vi "PH_gentec_M-Link.set Enable Anticipation.vi"(0 "i ref in":refnum<vi>, 2 "VISA resource in":refnum<visa-resource-name>, 5 "error in":errorcluster) -> (11 "Timeout":bool, 13 "Data read":string[](array[string]), 14 "i ref out":refnum<vi>, 16 "VISA resource out":refnum<visa-resource-name>, 17 "Error":bool, 18 "Failure":bool, 19 "error out":errorcluster)   [LabVIEW 2014, in "PH_gentec_M-Link.lvlib"]
doc: "This VI writes wanted Settings to the Device and checks the result."
uses:
  PH_gentec_M-Link.lvlib
  non_GPL/instr.lib/gentec-M-LINK/gentec-M-Link - Driver.lvlib
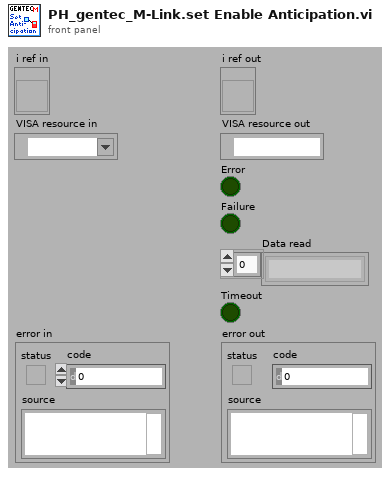
[diagram p1: front panel]
types:
  T1 = typedef "PH_gentec_M-Link.lvlib/PH_gentec_M-Link.i attribute.ctl" = cluster{"GUI References":cluster{"Wanted Head Settings":refnum<vi>, "Current Head Settings":refnum<vi>, "Set Auto Range":refnum<vi>, "Trigger Polarity":refnum<vi>, "Trigger Source":refnum<vi>, "Waveform Averages":refnum<vi>, "Continuous":refnum<vi>, "get one Value":refnum<vi>}, "Wanted Head Settings":T2, "Current Head Settings":T2}
  T2 = typedef "PH_gentec_M-Link.lvlib/PH_gentec_M-Link.Head Settings.ctl" = cluster{"Measurement Mode":T3, "Enable Anticipation":bool, "Set Auto Range":bool, "Block Signal":bool, "Set Head Attenuator":bool, "Enable SSE":bool, "Trigger Polarity":T4, "Trigger Source":T5, "Waveform Averages":T6, "Set Zero":i32, "Current Measurement":i32, "Start Data Flow":bool}
  T3 = typedef "gentec-M-Link - Driver.lvlib/gentec-M-Link.Measurement Mode.ctl" = u16
  T4 = typedef "gentec-M-Link - Driver.lvlib/gentec-M-Link.Trigger Polarity.ctl" = u16
  T5 = typedef "gentec-M-Link - Driver.lvlib/gentec-M-Link.Trigger Source.ctl" = u16
  T6 = typedef "gentec-M-Link - Driver.lvlib/gentec-M-Link.Waveform Averages.ctl" = u16
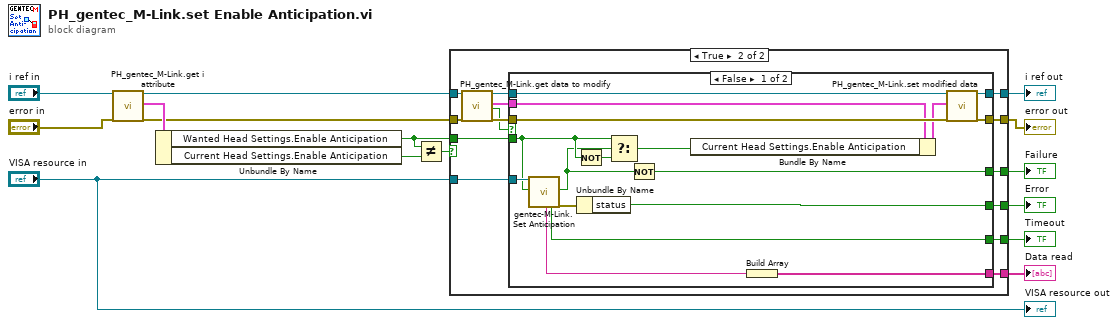
[diagram p0: block diagram]
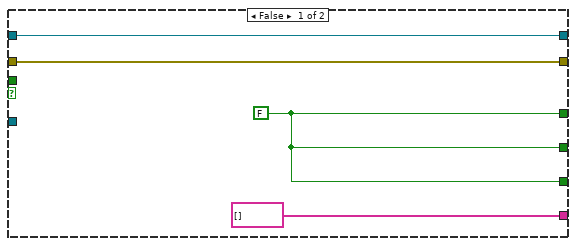
[diagram p2: hidden frame]
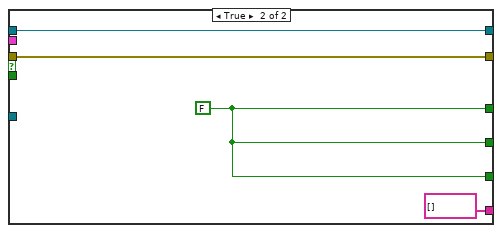
[diagram p3: hidden frame]
diagram:
  n1 = call "PH_gentec_M-Link.get i attribute.vi"("i ref in"="i ref in", "error in (no error)"="error in") -> ("i ref out"=w10:refnum<vi>, "i attribute"=w13:T1, "error out"=w12:errorcluster)  [unwired: 15 in]
  n2 = Unbundle By Name(w13) -> ("Wanted Head Settings.Enable Anticipation"=w6:bool, "Current Head Settings.Enable Anticipation"=w7:bool)
  n3 = Not Equal?(x=w6, y=w7) -> (x != y?=w5:bool)
  n4 = case shown="True" w5 {
    tunnel: [w18 w33] -> w15
    tunnel: [w19 w32] -> w14
    tunnel: w12 -> [w18 w27]
    tunnel: w10 -> [w19 w26]
    tunnel: "VISA resource in" -> [_ w25]
    tunnel: w6 -> [_ w24]
    tunnel: [w17 w23] -> w4
    tunnel: [w17 w22] -> w3
    tunnel: [w17 w21] -> w2
    tunnel: [string[] [] w20] -> w1
    frame False {
      w17 = FALSE
    }
    frame True {
      n5 = call "PH_gentec_M-Link.get data to modify.vi"("i ref in"=w26, "error in (no error)"=w27) -> ("i ref out"=w30:refnum<vi>, "i attribute"=w29:T1, "timed out"=w28:bool, "error out"=w31:errorcluster)  [unwired: 14 in]
      n6 = case shown="False" w28 {
        tunnel: w25 -> [w49 _]
        tunnel: [w45 w54] -> w32
        tunnel: [w44 w53] -> w33
        tunnel: w31 -> [w48 w53]
        tunnel: w30 -> [w50 w54]
        tunnel: w29 -> [w39 _]
        tunnel: w24 -> [w46 _]
        tunnel: [w38 w52] -> w23
        tunnel: [w37 w52] -> w22
        tunnel: [w36 w52] -> w21
        tunnel: [w34 string[] []] -> w20
        frame False {
          n7 = call "gentec-M-Link.Set Anticipation.vi"("VISA resource In"=w49, "Enable Anticipation"=w46) -> ("Data Read"=w35:string, "Read Timeout"=w36:bool, "Success"=w42:bool, "error out"=w43:errorcluster)  [unwired: 13 in, 1 out]
          n8 = Not(x=w46) -> (.not. x?=w41:bool)
          n9 = Unbundle By Name(w43) -> ("status"=w38:bool)
          n10 = Select(t=w46, s=w42, f=w41) -> (s? t:f=w40:bool)
          n11 = Not(x=w42) -> (.not. x?=w37:bool)
          n12 = Bundle By Name(cluster=w39, "Current Head Settings.Enable Anticipation"=w40) -> (w47:T1)
          n13 = Build Array(w35) -> (w34:string[])
          n14 = call "PH_gentec_M-Link.set modified data.vi"("i ref in"=w50, "i attribute"=w47, "error in (no error)"=w48) -> ("i ref out"=w45:refnum<vi>, "error out"=w44:errorcluster)  [unwired: 15 in]
        }
        frame True {
          w52 = FALSE
        }
      }
    }
  }
  "error out" <- w15
  "i ref out" <- w14
  "Data read" <- w1
  "Timeout" <- w2
  "Error" <- w4
  "Failure" <- w3
  "VISA resource out" <- "VISA resource in"
